vi "Integer Check Columns.vi"(11 "Sudoku Int":u8[][](array[numeric])) -> (3 "Is Ok":bool)   [LabVIEW 2015, in "Sudoku Library.lvlib"]
doc: "Created IvanLis by LabVIEW Portal\nProfile: http://labviewportal.org/memberlist.php?mode=viewprofile&u=987\neMail: IvanLisanov@gMail.com\nTelegram: https://t.me/IvanLis"
uses:
  Sudoku Library.lvlib
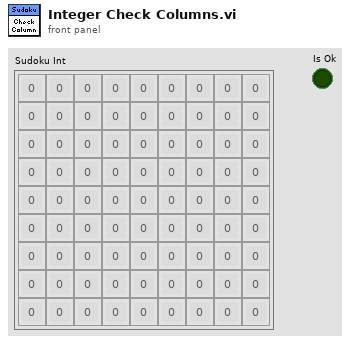
[diagram p1: front panel]
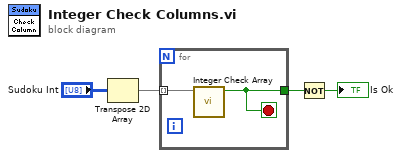
[diagram p0: block diagram]
diagram:
  n1 = Transpose 2D Array(2D array="Sudoku Int") -> (transposed array=w1:u8[][])
  n2 = for {
    tunnel: w1 -> [w6] mode=indexing
    tunnel: [w5] -> w3
    stop <- w5 stop-if-true
    n3 = call "Integer Check Array.vi"("Array"=w6) -> ("Error"=w5:bool)  [unwired: 10 in]
  }
  n4 = Not(x=w3) -> (.not. x?=→"Is Ok":bool)
